vi "Write DC.vi"(8 "error in (no error)":errorcluster, 10 "Rate (Hz)":dbl, 11 "Change Blue Laser Rate MSG in":refnum<class "Change Blue DC MSG.lvclass">) -> (0 "error out":errorcluster, 3 "Change Blue Laser Rate MSG out":refnum<class "Change Blue DC MSG.lvclass">)   [LabVIEW 2014, in "eCRDS Library.lvlib" / "Change Blue DC MSG.lvclass"]
uses:
  Change Blue DC MSG.lvclass
  Change Blue DC MSG.lvclass/Change Blue DC MSG.ctl
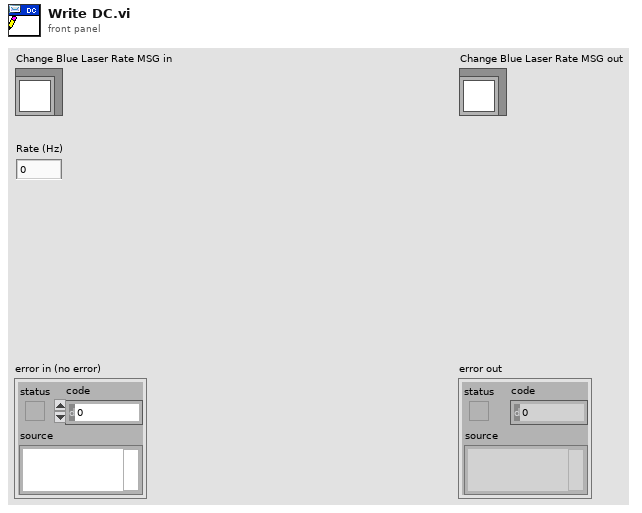
[diagram p1: front panel]
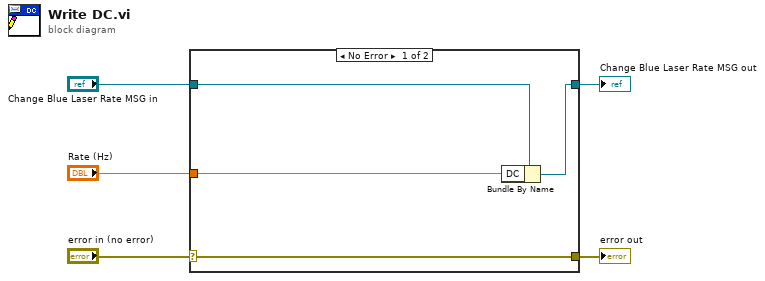
[diagram p0: block diagram]
diagram:
  n1 = case shown="No Error" "error in (no error)" {
    selector: "error in (no error)" -> [w9 w10]
    tunnel: [w9 w10] -> w4
    tunnel: [w7 w11] -> w2
    tunnel: "Change Blue Laser Rate MSG in" -> [w8 w11]
    tunnel: "Rate (Hz)" -> [w6 _]
    frame No Error {
      n2 = Bundle By Name(cluster=w8, "DC"=w6) -> (w7:refnum<class "Change Blue DC MSG.lvclass">)
    }
    frame Error {
    }
  }
  "error out" <- w4
  "Change Blue Laser Rate MSG out" <- w2
